vi "Compute DistanceToBalls.vi"(6 "Target Width (in)":dbl=6.0 format="%#_13g", 8 "results":T1, 11 "Image Src":T2) -> (0 "results out":T1, 3 "Image Dst Out":T2)   [LabVIEW 2019]
doc: "Using the camera lens information and the real world size of the target, use trig and ratios to determine the distance to the target. Also returns the location relative to the image center in a (-1 , 1) coordinate system that may be useful for steering the robot."
uses:
  <vilib>/vision/Image Controls.llb/IMAQ Image.ctl
  Target Fields.ctl
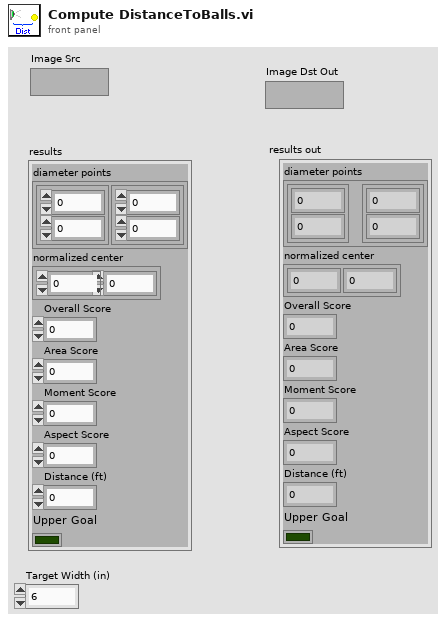
[diagram p1: front panel]
types:
  T1 = typedef "Target Fields.ctl" = cluster{"diameter points":cluster{"first point":cluster{"x":dbl, "y":dbl}, "projected point":cluster{"x":dbl, "y":dbl}}, "normalized center":cluster{"x":dbl, "y":dbl}, "Overall Score":dbl, "Area Score":dbl, "Moment Score":dbl, "Aspect Score":dbl, "Distance (ft)":dbl, "Upper Goal":bool}
  T2 = typedef "IMAQ Image.ctl" = refnum<image>
  T3 = cluster{"first point":cluster{"x":dbl, "y":dbl}, "projected point":cluster{"x":dbl, "y":dbl}}
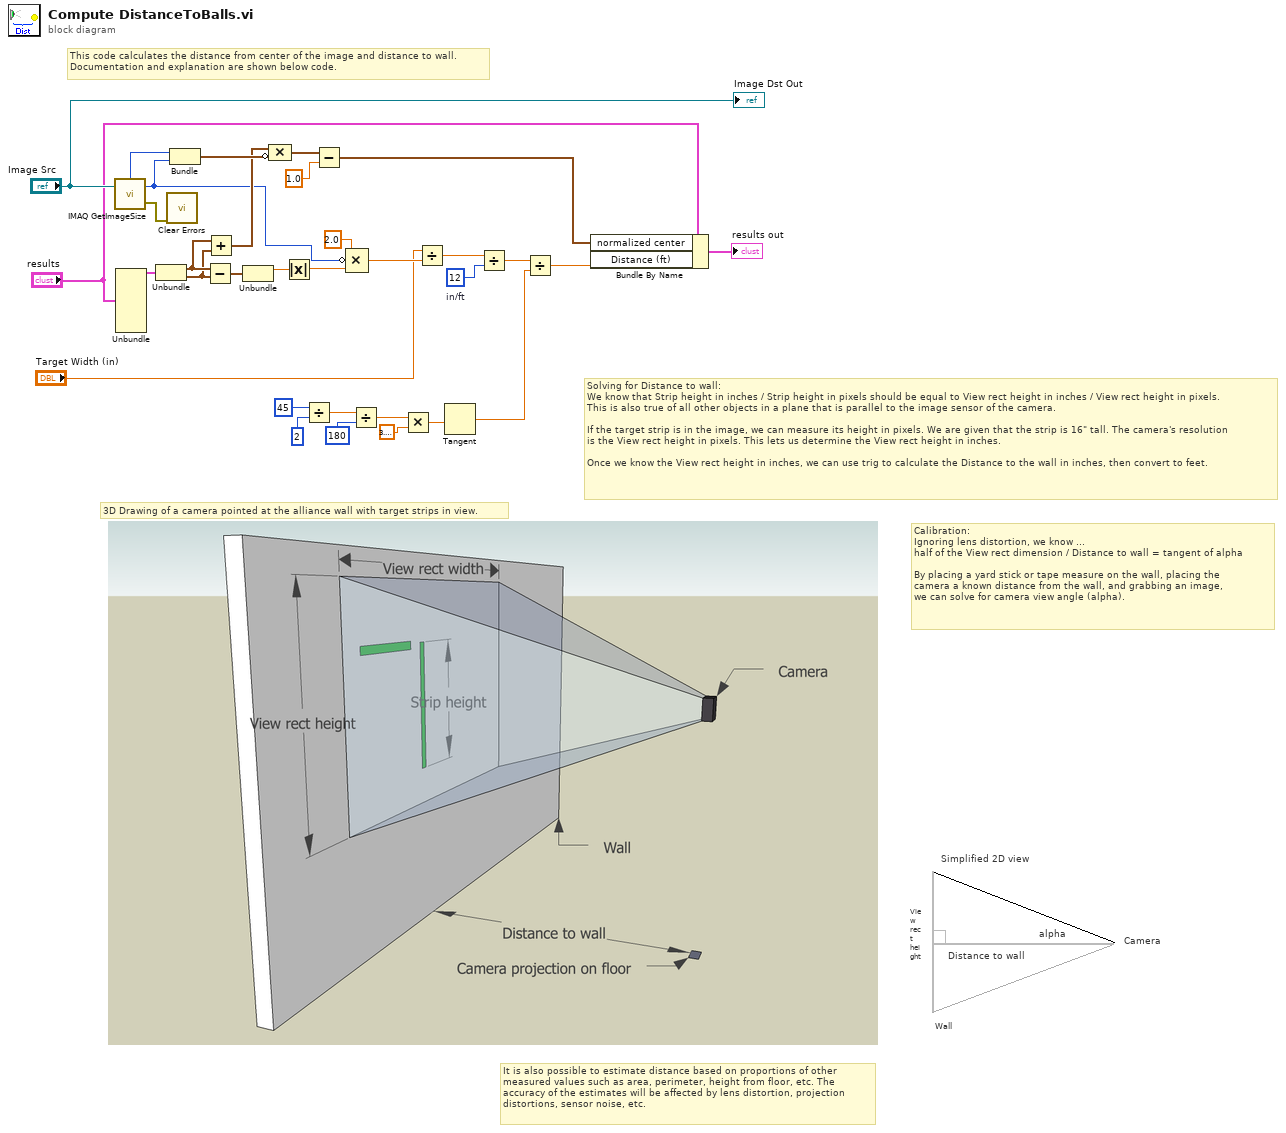
[diagram p0: block diagram]
diagram:
  w32 = 12  # in/ft
  # "It is also possible to estimate distance based on proportions of other\nmeasured values such as area, perimeter, height from floor, etc. The\naccuracy of the estimates will be affected by lens distortion, projection\ndistortions, sensor noise, etc."
  # "Wall"
  # "Camera"
  # "Simplified 2D view"
  # "Solving for Distance to wall:\nWe know that Strip height in inches / Strip height in pixels should be equal to View rect height in inches / View rect height in pixels.\nThis is also true of all other objects in a plane that is parallel to the image sensor of the camera.\n\nIf the target strip is in the image, we can measure its height in pixels. We are given that the strip is 16\" tall. The camera's resolution\nis the View rect height in pixels. This lets us determine the View rect height in inches.\n\nOnce we know the View rect height in inches, we can use trig to calculate the Distance to the wall in inches, then convert to feet."
  # "3D Drawing of a camera pointed at the alliance wall with target strips in view."
  # "Distance to wall"
  # "View rect height"
  # "alpha"
  # "Calibration:\nIgnoring lens distortion, we know ...\nhalf of the View rect dimension / Distance to wall = tangent of alpha\n\nBy placing a yard stick or tape measure on the wall, placing the\ncamera a known distance from the wall, and grabbing an image,\nwe can solve for camera view angle (alpha)."
  # "This code calculates the distance from center of the image and distance to wall.\nDocumentation and explanation are shown below code."
  n1 = call "IMAQ GetImageSize"("Image"="Image Src") -> ("Y Resolution"=w10:i32, "X Resolution"=w19:i32, "error out"=w28:errorcluster)  [unwired: 3 in]
  n2 = Unbundle("results") -> ("diameter points"=w18:T3)  [unwired: 7 out]
  n3 = Unbundle(w18) -> ("first point"=w14:cluster{"x":dbl, "y":dbl}, "projected point"=w13:cluster{"x":dbl, "y":dbl})
  n4 = call <vilib>:"Clear Errors.vi"("error in (no error)"=w28) -> ()  [unwired: 5 in, 2 out]
  n5 = Bundle("X Resolution"=w19, "Y Resolution"=w10) -> (w15:cluster{"X Resolution":i32, "Y Resolution":i32})  [unwired: 1 in]
  n6 = Subtract(x=w14, y=w13) -> (x-y=w24:cluster{"x":dbl, "y":dbl})
  n7 = Add(x=w14, y=w13) -> (x+y=w12:cluster{"x":dbl, "y":dbl})
  n8 = Unbundle(w24) -> ("x"=w23:dbl)  [unwired: 1 out]
  n9 = Compound Arithmetic op=MULTIPLY(w12, invert w15) -> (w17:cluster{dbl, dbl})
  n10 = Absolute Value(x=w23) -> (abs(x)=w25:dbl)
  n11 = Divide(x=45, y=2) -> (x/y=w5:dbl)
  n12 = Subtract(x=w17, y=1.0) -> (x-y=w16:cluster{dbl, dbl})
  n13 = Compound Arithmetic op=MULTIPLY(2.0, invert w10, w25) -> (w29:dbl)
  n14 = Divide(x=w5, y=180) -> (x/y=w4:dbl)
  n15 = Multiply(x=w4, y=3.141592653589793) -> (x*y=w6:dbl)
  n16 = Divide(x="Target Width (in)", y=w29) -> (x/y=w26:dbl)
  n17 = Tangent(1:w6) -> (0:w1:dbl)
  n18 = Divide(x=w26, y=w32) -> (x/y=w31:dbl)
  n19 = Divide(x=w31, y=w1) -> (x/y=w20:dbl)
  n20 = Bundle By Name(cluster="results", "normalized center"=w16, "Distance (ft)"=w20) -> (→"results out":T1)
  "Image Dst Out" <- "Image Src"
